vi "GetFileNortekFTP.vi"(4 "error in (no error)":errorcluster caption="entrée d'erreur (pas d'erreur)", 6 "NewNortekFile":path) -> (0 "error out":errorcluster caption="sortie d'erreur", 2 "FichierNortek":path)   [LabVIEW 2017]
uses:
  <vilib>/FTP/NI_FTP.lvlib
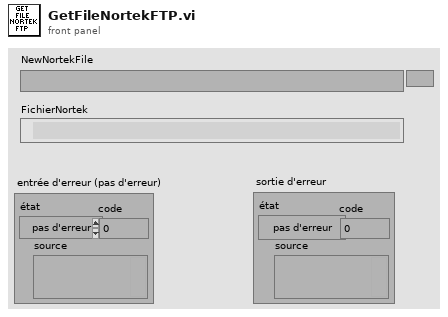
[diagram p1: front panel]
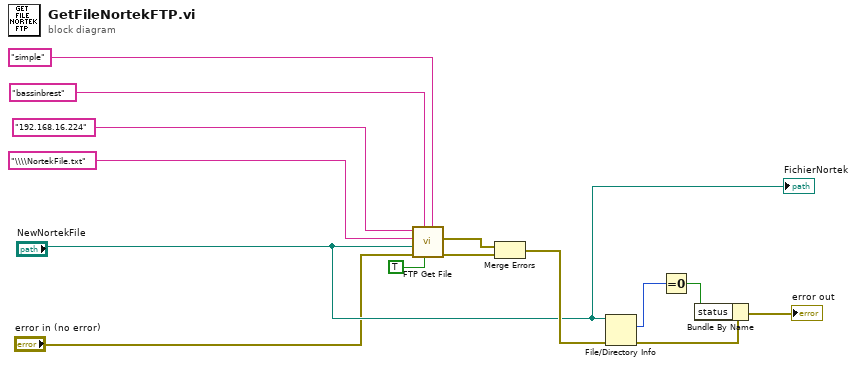
[diagram p0: block diagram]
diagram:
  n1 = call <vilib>:"FTP Get File.vi"("password"="simple", "binary (F)"=TRUE, "user"="bassinbrest", "error in (no error)"="error in (no error)", "local path"="NewNortekFile", "remote path"="\\\\NortekFile.txt" ("chaîne"), "host"="192.168.16.224" ("NortekPC-IPadress")) -> ("error out"=w9:errorcluster, "file error"=w10:errorcluster)  [unwired: 3 in]
  n2 = Merge Errors(w10, w9) -> (w8:errorcluster)
  n3 = File/Directory Info(path="NewNortekFile", error in=w8) -> (size=w7:i64, error out=w4:errorcluster)  [unwired: 5 out]
  n4 = Equal To 0?(x=w7) -> (x = 0?=w6:bool)
  n5 = Bundle By Name(cluster=w4, "status"=w6) -> (→"error out":errorcluster)
  "FichierNortek" <- "NewNortekFile"
